vi "CvrtCell2Data.vi"(8 "error in (no error)":errorcluster, 9 "ge_HdrNames":T1, 10 "Item Name":string, 11 "Dynamic.lvclass":refnum<class "Dynamic.lvclass">) -> (0 "error out":errorcluster, 3 "Dynamic out":refnum<class "Dynamic.lvclass">)   [LabVIEW 2012, in "Measurement Channels.lvlib" / "Dynamic.lvclass"]
uses:
  Dynamic.lvclass
  Common/Controls/HeaderNames.ctl
  Class Voltage/Voltage.lvclass
  Dynamic.lvclass/Dynamic.ctl
  SubVIs Table/Custom Ctls Table/ge_ColType.ctl
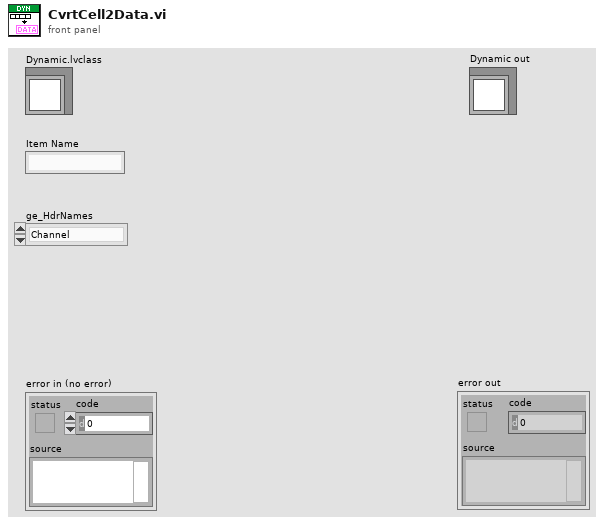
[diagram p1: front panel]
types:
  T1 = typedef "HeaderNames.ctl" = enum16{"Channel", "Device", "Spacer", "Description", "MB", "Range", "Terminal", "Coupling", "Thresh (V)", "Pulse/Rev", "Slope", "Min EU", "Min RPM", "mV/EU", "Iex", "Temp Units", "Type", "CJC Src", "CJC Val", "Ro", "Wire Cfg", "Strain Mode", "Vex", "Bridge Type", "GF", "Gauge Res", "Poisson", "Lead Res", "Init Strain", "GAF", "Scale", "Offset", "Unit (EU)", "dB?", "dB Ref", "Cal Mag", "Cal Units", "Max Temp", "Min Temp", "Max Strain", "Min Strain"}
  T2 = typedef "ge_ColType.ctl" = enum16{"Volts", "Amps", "Ohms", "TermCfg", "WireCfg", "Coup", "Slope", "Iex", "CalUnits", "ThrmUnits", "ThrmType", "CJCSrc", "BrdgType", "Strn Mode", "RTDType"}
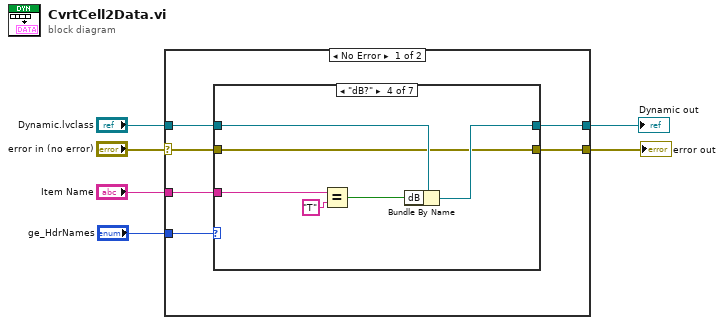
[diagram p0: block diagram]
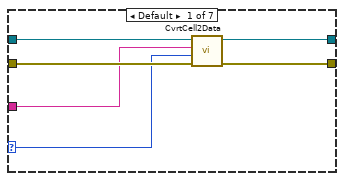
[diagram p2: hidden frame]
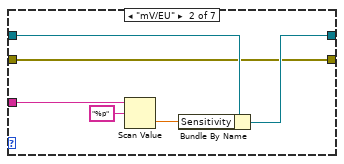
[diagram p3: hidden frame]
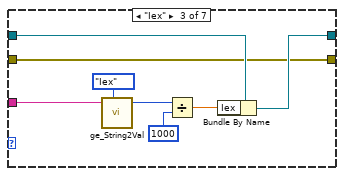
[diagram p4: hidden frame]
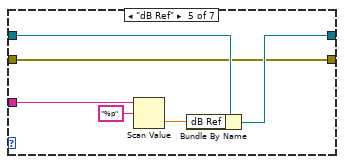
[diagram p5: hidden frame]
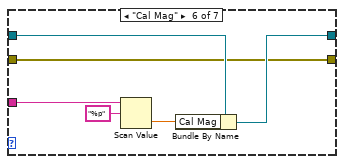
[diagram p6: hidden frame]
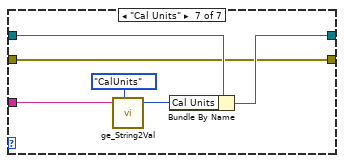
[diagram p7: hidden frame]
diagram:
  n1 = case shown="No Error" "error in (no error)" {
    selector: "error in (no error)" -> [w7 w57]
    tunnel: [w12 w58] -> w6
    tunnel: "Item Name" -> [w11 _]
    tunnel: "ge_HdrNames" -> [w10 _]
    tunnel: "Dynamic.lvclass" -> [w9 w58]
    tunnel: [w8 w57] -> w2
    frame No Error {
      n2 = case shown="\"dB?\"" w10 {
        selector: w10 -> [w13 _ _ _ _ _ _]
        tunnel: w11 -> [w14 w20 w31 w37 w40 w46 w54]
        tunnel: w9 -> [w18 w24 w30 w35 w44 w50 w56]
        tunnel: [w17 w23 w29 w34 w43 w49 w52] -> w12
        tunnel: w7 -> [w16 w22 w25 w33 w42 w48 w51]
        tunnel: [w15 w22 w25 w33 w42 w48 w51] -> w8
        frame Default {
          n3 = call-parent "CvrtCell2Data.vi"("error in"=w16, "ge_HdrNames"=w13, "Item Name"=w14, "Voltage In"=w18) -> ("error out"=w15:errorcluster, "Voltage Out"=w17:refnum<class "Dynamic.lvclass">)  [unwired: 6 in]
        }
        frame "mV/EU" {
          n4 = Scan Value(string=w20, format string="%p") -> (value=w19:dbl)  [unwired: 1 in, 1 out]
          n5 = Bundle By Name(cluster=w24, "Sensitivity"=w19) -> (w23:refnum<class "Dynamic.lvclass">)
        }
        frame "Iex" {
          n6 = call "ge_String2Val.vi"("String"=w31, "ColType"=ge_ColType."Iex") -> ("Value"=w27:u16)  [unwired: 4 in, 1 out]
          n7 = Divide(x=w27, y=1000) -> (x/y=w26:dbl)
          n8 = Bundle By Name(cluster=w30, "Iex"=w26) -> (w29:refnum<class "Dynamic.lvclass">)
        }
        frame "dB?" {
          n9 = Equal?(x=w37, y="T") -> (x = y?=w36:bool)
          n10 = Bundle By Name(cluster=w35, "dB"=w36) -> (w34:refnum<class "Dynamic.lvclass">)
        }
        frame "dB Ref" {
          n11 = Scan Value(string=w40, format string="%p") -> (value=w39:dbl)  [unwired: 1 in, 1 out]
          n12 = Bundle By Name(cluster=w44, "dB Ref"=w39) -> (w43:refnum<class "Dynamic.lvclass">)
        }
        frame "Cal Mag" {
          n13 = Scan Value(string=w46, format string="%p") -> (value=w45:dbl)  [unwired: 1 in, 1 out]
          n14 = Bundle By Name(cluster=w50, "Cal Mag"=w45) -> (w49:refnum<class "Dynamic.lvclass">)
        }
        frame "Cal Units" {
          n15 = call "ge_String2Val.vi"("String"=w54, "ColType"=ge_ColType."CalUnits") -> ("Value"=w53:u16)  [unwired: 4 in, 1 out]
          n16 = Bundle By Name(cluster=w56, "Cal Units"=w53) -> (w52:refnum<class "Dynamic.lvclass">)
        }
      }
    }
    frame Error {
    }
  }
  "error out" <- w2
  "Dynamic out" <- w6
